vi "write voltage.vi"(10 "Voltage":dbl, 11 "Display Panel.lvlib:Write Voltage Msg.lvclass":refnum<class "Write Voltage Msg.lvclass">) -> (3 "Display Panel.lvlib:Write Voltage Msg.lvclass 2":refnum<class "Write Voltage Msg.lvclass">)   [LabVIEW 2016, in "Display Panel.lvlib" / "Write Voltage Msg.lvclass"]
uses:
  Write Voltage Msg.lvclass
  Write Voltage Msg.lvclass/Write Voltage Msg.ctl
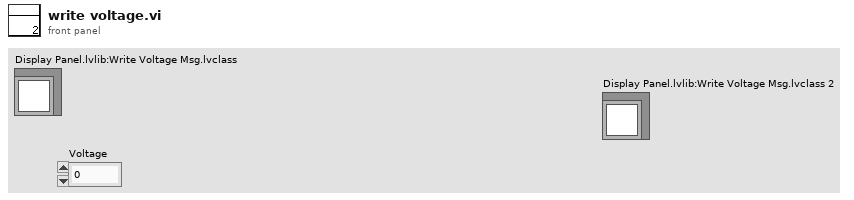
[diagram p1: front panel]
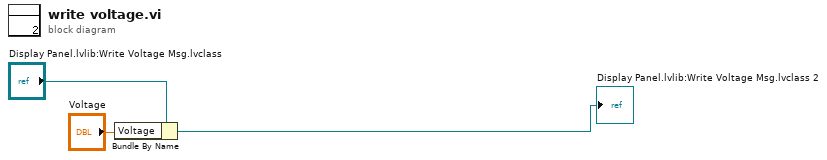
[diagram p0: block diagram]
diagram:
  n1 = Bundle By Name(cluster="Display Panel.lvlib:Write Voltage Msg.lvclass", "Voltage"="Voltage") -> (→"Display Panel.lvlib:Write Voltage Msg.lvclass 2":refnum<class "Write Voltage Msg.lvclass">)
